vi "run.vi"(8 "error in (no error)":errorcluster, 11 "DataCollectionDL091104Scaffold.lvclass out":refnum<class "DataCollectionDL091104Scaffold.lvclass">) -> (0 "error out":errorcluster, 3 "DataCollectionDL091104Scaffold.lvclass out":refnum<class "DataCollectionDL091104Scaffold.lvclass">)   [LabVIEW 2010, in "DataCollectionDL091104Scaffold.lvclass"]
uses:
  DataCollectionDL091104Scaffold.lvclass
  action_enum.ctl
  DataCollectionDL091104Scaffold.lvclass/DataCollectionDL091104Scaffold.ctl
  GenericDataCollection/GenericDataCollection/GenericDataCollection.lvclass
  common/classes/ErrorController/ErrorController/class_data.vi
  common/classes/ErrorController/ErrorController/ErrorController.lvclass
panel:
  out "last action":T1=enum."initialise"
  out "event loop counter":i32
  out "statechart loop counter":i32=49
  out "error":errorcluster
  in  "play movie?":bool
  out "finished?":bool=TRUE
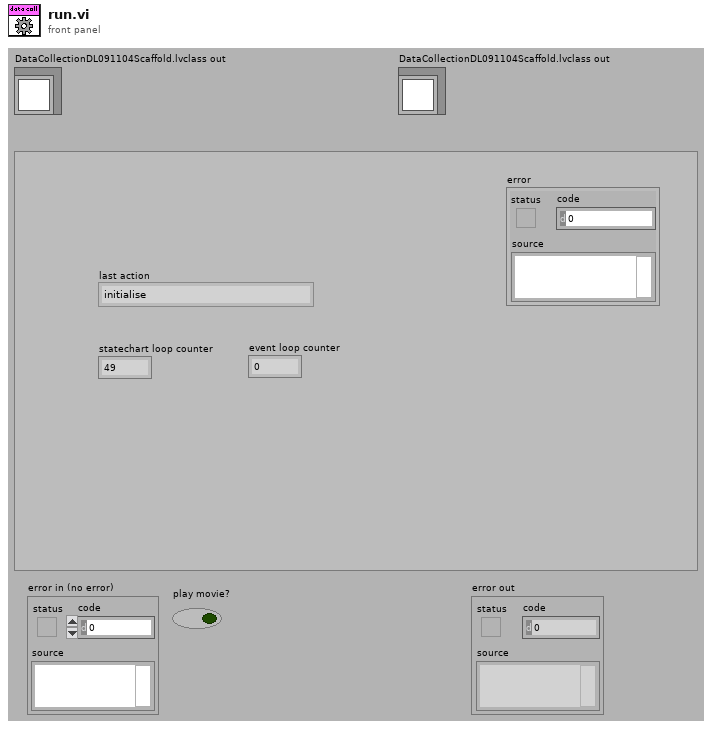
[diagram p1: front panel]
types:
  T1 = typedef "DataCollectionDL091104Scaffold.lvclass/action_enum.ctl" = enum16{"NULL", "initialise", "terminate", "reset", "insert", "save", "register as observer", "sweep finished", "attach observer", "detach observer"}
  T2 = typedef "top-level_component_type_enum.ctl" = enum16{"undefined", "ImagingMode", "ScanHead", "DAQ", "ImageAssembler", "Display", "DataCollection", "Analyser", "Stimulator", "ExperimentController", "Instrument", "Stage"}
  T3 = typedef "main_trigger_enum.ctl" = enum16{"NULL", "initialise", "terminate", "start", "stop", "change objective", "change experimentController", "change imagingMode", "save notebook", "started saving", "finished saving", "expCtr ready", "expCtr missing", "imgMd ready", "imgMd missing", "scanHd ready", "scanHd missing", "DAQ ready", "DAQ missing", "imgAsm ready", "imgAsm missing", "dataColl ready", "dataColl missing", "display ready", "display missing", "analysr ready", "analysr missing", "instrmnt ready", "instrmnt missing", "stimltr ready", "stimltr missing", "stage ready", "stage missing"}
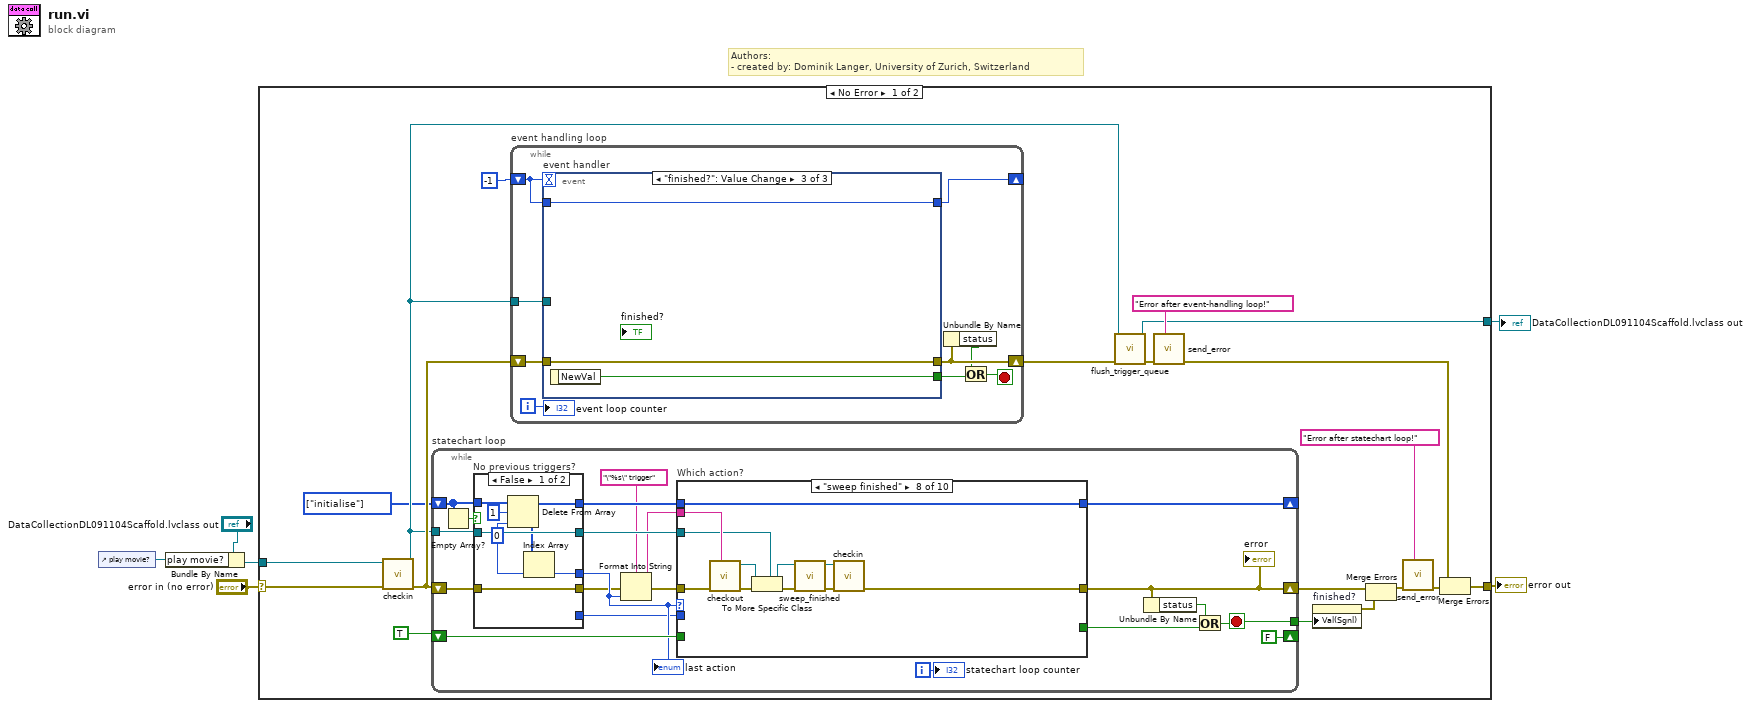
[diagram p0: block diagram]
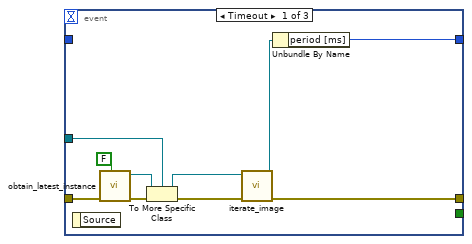
[diagram p2: hidden frame]
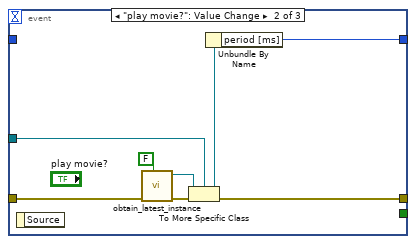
[diagram p3: hidden frame]
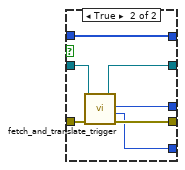
[diagram p4: hidden frame]
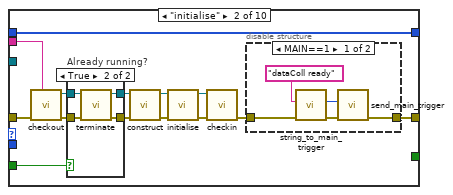
[diagram p6: hidden frame]
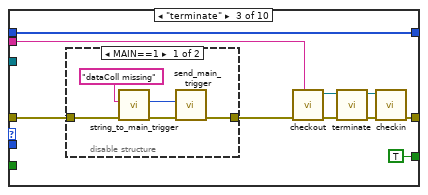
[diagram p9: hidden frame]
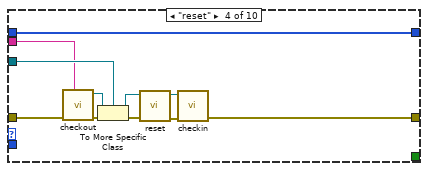
[diagram p11: hidden frame]
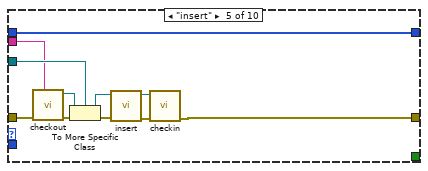
[diagram p12: hidden frame]
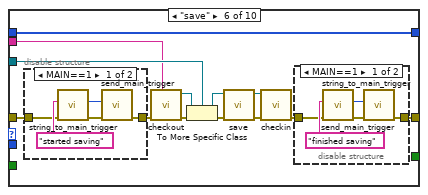
[diagram p13: hidden frame]
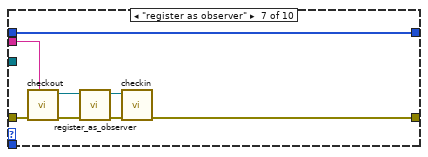
[diagram p16: hidden frame]
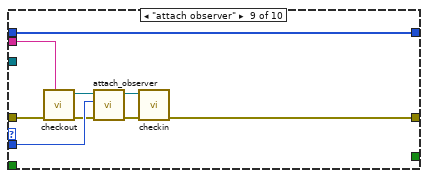
[diagram p17: hidden frame]
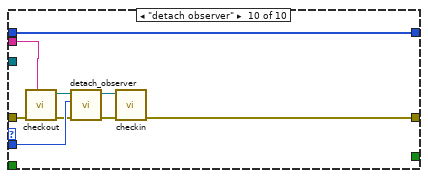
[diagram p18: hidden frame]
diagram:
  # "Authors: \n- created by: Dominik Langer, University of Zurich, Switzerland"
  n1 = control-ref of="play movie?"() -> (w3:refnum<vi>)
  n2 = Bundle By Name(cluster="DataCollectionDL091104Scaffold.lvclass out", "play movie?"=w3) -> (w4:refnum<class "DataCollectionDL091104Scaffold.lvclass">)
  n3 = case shown="No Error" "error in (no error)" {
    selector: "error in (no error)" -> [w7 w220]
    tunnel: [w20 w220] -> w5
    tunnel: [w13 w219] -> w2
    tunnel: w4 -> [w8 w219]
    frame No Error {
      w9 = T1[] [enum."initialise"] items=["NULL", "initialise", "terminate", "reset", "insert", "save", "register as observer", "sweep finished", "attach observer", "detach observer"]
      n4 = call-dynamic "checkin.vi"("error in (no error)"=w7, "GenericDataCollection in"=w8) -> ("error out"=w17:errorcluster, "GenericDataCollection out"=w14:refnum<class "DataCollectionDL091104Scaffold.lvclass">)  [unwired: 8 in]
      n5 = while "statechart loop" {
        shift-right: [FALSE] -> _
        shift-left: TRUE -> [w68]
        tunnel: [w66] -> w23
        tunnel: w14 -> [w73]
        shift-right: [w71] -> w11
        shift-left: w17 -> [w72]
        shift-right: [w62] -> _
        shift-left: w9 -> [w65]
        i -> [w75]
        stop <- w66 stop-if-true
        n6 = Empty Array?(array=w65) -> (empty?=w64:bool)
        n7 = case "No previous triggers?" shown="False" w64 {
          tunnel: w73 -> [w81 w90]
          tunnel: w72 -> [w79 w89]
          tunnel: [w79 w88] -> w59
          tunnel: [w81 w87] -> w67
          tunnel: [w80 w86] -> w61
          tunnel: w65 -> [w83 w85]
          tunnel: [w77 w85] -> w63
          tunnel: [_ w84] -> w56
          frame False {
            w76 = 0 ("index")
            n8 = Delete From Array(array=w83, length=1, index=w76) -> (deleted portion=w78:T1[], array with subset deleted=w77:T1[])
            n9 = Index Array(array=w78, index=w76) -> (element=w80:T1)
          }
          frame True {
            n10 = call-dynamic "fetch_and_translate_trigger.vi"("error in (no error)"=w89, "DataCollectionDL091104Scaffold in"=w90) -> ("error out"=w88:errorcluster, "sender TLC type"=w84:T2, "trigger"=w86:T1, "DataCollectionDL091104Scaffold out"=w87:refnum<class "DataCollectionDL091104Scaffold.lvclass">)  [unwired: 6 in]
          }
        }
        "last action" <- w61
        n11 = Format Into String(format string="\"%s\" trigger", error in=w59, w61) -> (resulting string=w58:string, error out=w60:errorcluster)  [unwired: 1 in]
        n12 = case "Which action?" shown="\"sweep finished\"" w61 {
          tunnel: w60 -> [w92 w98 w122 w145 w149 w160 w187 w197 w207 w216]
          tunnel: [w92 w95 w123 w144 w148 w157 w186 w196 w204 w211] -> w71
          tunnel: [_ _ TRUE _ _ _ _ _ _ _] -> w69
          tunnel: w68 -> [_ w97 _ _ _ _ _ _ _ _]
          tunnel: w67 -> [_ _ _ w143 w150 w163 _ w194 _ _]
          tunnel: w63 -> [w91 w94 w120 w142 w147 w162 w183 w200 w209 w218]
          tunnel: [w91 w94 w120 w142 w147 w162 w183 w200 w209 w218] -> w62
          tunnel: w58 -> [_ w93 w119 w141 w146 w161 w182 w195 w201 w213]
          tunnel: w56 -> [_ _ _ _ _ _ _ _ w208 w217]
          frame "NULL", Default {
          }
          frame "initialise" {
            n13 = call "checkout.vi"("locked by?"=w93, "error in (no error)"=w98) -> ("error out"=w105:errorcluster, "GenericDataCollection out"=w103:refnum<class "GenericDataCollection.lvclass">)  [unwired: 8 in]
            n14 = case "Already running?" shown="True" w97 {
              tunnel: [w114 w118] -> w106
              tunnel: w105 -> [w114 w117]
              tunnel: [w113 w116] -> w104
              tunnel: w103 -> [w113 w115]
              frame False {
              }
              frame True {
                n15 = call-dynamic "terminate.vi"("error in (no error)"=w117, "GenericPlugin in"=w115) -> ("error out"=w118:errorcluster, "GenericPlugin out"=w116:refnum<class "GenericDataCollection.lvclass">)  [unwired: 8 in]
              }
            }
            n16 = call-dynamic "construct.vi"("error in (no error)"=w106, "GenericPlugin in"=w104) -> ("error out"=w101:errorcluster, "GenericPlugin out"=w100:refnum<class "GenericDataCollection.lvclass">)  [unwired: 8 in]
            n17 = call-dynamic "initialise.vi"("error in (no error)"=w101, "GenericPlugin in"=w100) -> ("error out"=w102:errorcluster, "GenericPlugin out"=w99:refnum<class "GenericDataCollection.lvclass">)  [unwired: 8 in]
            n18 = call-dynamic "checkin.vi"("error in (no error)"=w102, "GenericDataCollection in"=w99) -> ("error out"=w96:errorcluster)  [unwired: 8 in, 1 out]
            n19 = disable-structure shown="MAIN==1" {
              disable-tunnel: w96 -> [w109 w112]
              disable-tunnel: [w111 w112] -> w95
              frame condition #0 (active) {
                n20 = call "string_to_main_trigger.vi"("error in (no error)"=w109, "trigger string"="dataColl ready") -> ("error out"=w108:errorcluster, "main trigger"=w107:T3)  [unwired: 8 in]
                n21 = call "send_main_trigger.vi"("error in (no error)"=w108, "trigger"=w107) -> ("error out"=w111:errorcluster)  [unwired: 9 in]
              }
              frame condition #1 {
              }
            }
          }
          frame "terminate" {
            n22 = disable-structure shown="MAIN==1" {
              disable-tunnel: w122 -> [w131 w134]
              disable-tunnel: [w133 w134] -> w121
              frame condition #0 (active) {
                n23 = call "string_to_main_trigger.vi"("error in (no error)"=w131, "trigger string"="dataColl missing") -> ("error out"=w130:errorcluster, "main trigger"=w129:T3)  [unwired: 8 in]
                n24 = call "send_main_trigger.vi"("error in (no error)"=w130, "trigger"=w129) -> ("error out"=w133:errorcluster)  [unwired: 9 in]
              }
              frame condition #1 {
              }
            }
            n25 = call "checkout.vi"("locked by?"=w119, "error in (no error)"=w121) -> ("error out"=w127:errorcluster, "GenericDataCollection out"=w125:refnum<class "GenericDataCollection.lvclass">)  [unwired: 8 in]
            n26 = call-dynamic "terminate.vi"("error in (no error)"=w127, "GenericPlugin in"=w125) -> ("error out"=w126:errorcluster, "GenericPlugin out"=w124:refnum<class "GenericDataCollection.lvclass">)  [unwired: 8 in]
            n27 = call-dynamic "checkin.vi"("error in (no error)"=w126, "GenericDataCollection in"=w124) -> ("error out"=w123:errorcluster)  [unwired: 8 in, 1 out]
          }
          frame "reset" {
            n28 = call "checkout.vi"("locked by?"=w141, "error in (no error)"=w145) -> ("error out"=w137:errorcluster, "GenericDataCollection out"=w140:refnum<class "GenericDataCollection.lvclass">)  [unwired: 8 out]
            n29 = To More Specific Class(target class=w143, reference=w140, error in=w137) -> (specific class reference=w139:refnum<class "DataCollectionDL091104Scaffold.lvclass">, error out=w136:errorcluster)
            n30 = call-dynamic "reset.vi"("error in (no error)"=w136, "DataCollectionDL091104Scaffold in"=w139) -> ("error out"=w135:errorcluster, "DataCollectionDL091104Scaffold out"=w138:refnum<class "DataCollectionDL091104Scaffold.lvclass">)  [unwired: 8 in]
            n31 = call-dynamic "checkin.vi"("error in (no error)"=w135, "GenericDataCollection in"=w138) -> ("error out"=w144:errorcluster)  [unwired: 8 in, 1 out]
          }
          frame "insert" {
            n32 = call "checkout.vi"("locked by?"=w146, "error in (no error)"=w149) -> ("error out"=w155:errorcluster, "GenericDataCollection out"=w156:refnum<class "GenericDataCollection.lvclass">)  [unwired: 8 out]
            n33 = To More Specific Class(target class=w150, reference=w156, error in=w155) -> (specific class reference=w153:refnum<class "DataCollectionDL091104Scaffold.lvclass">, error out=w154:errorcluster)
            n34 = call-dynamic "insert.vi"("error in (no error)"=w154, "DL090215DataCollection in"=w153) -> ("error out"=w152:errorcluster, "DL090215DataCollection out"=w151:refnum<class "DataCollectionDL091104Scaffold.lvclass">)  [unwired: 8 out]
            n35 = call-dynamic "checkin.vi"("error in (no error)"=w152, "GenericDataCollection in"=w151) -> ("error out"=w148:errorcluster)  [unwired: 8 in, 1 out]
          }
          frame "save" {
            n36 = disable-structure shown="MAIN==1" {
              disable-tunnel: w160 -> [w178 w181]
              disable-tunnel: [w180 w181] -> w159
              frame condition #0 (active) {
                n37 = call "string_to_main_trigger.vi"("error in (no error)"=w178, "trigger string"="started saving") -> ("error out"=w177:errorcluster, "main trigger"=w176:T3)  [unwired: 8 in]
                n38 = call "send_main_trigger.vi"("error in (no error)"=w177, "trigger"=w176) -> ("error out"=w180:errorcluster)  [unwired: 9 in]
              }
              frame condition #1 {
              }
            }
            n39 = call "checkout.vi"("locked by?"=w161, "error in (no error)"=w159) -> ("error out"=w166:errorcluster, "GenericDataCollection out"=w169:refnum<class "GenericDataCollection.lvclass">)  [unwired: 8 out]
            n40 = To More Specific Class(target class=w163, reference=w169, error in=w166) -> (specific class reference=w167:refnum<class "DataCollectionDL091104Scaffold.lvclass">, error out=w165:errorcluster)
            n41 = call-dynamic "save.vi"("error in (no error)"=w165, "DL090215DataCollection in"=w167) -> ("error out"=w164:errorcluster, "DL090215DataCollection out"=w168:refnum<class "DataCollectionDL091104Scaffold.lvclass">)  [unwired: 8 out]
            n42 = call-dynamic "checkin.vi"("error in (no error)"=w164, "GenericDataCollection in"=w168) -> ("error out"=w158:errorcluster)  [unwired: 8 in, 1 out]
            n43 = disable-structure shown="MAIN==1" {
              disable-tunnel: w158 -> [w172 w175]
              disable-tunnel: [w174 w175] -> w157
              frame condition #0 (active) {
                n44 = call "string_to_main_trigger.vi"("error in (no error)"=w172, "trigger string"="finished saving") -> ("error out"=w171:errorcluster, "main trigger"=w170:T3)  [unwired: 8 in]
                n45 = call "send_main_trigger.vi"("error in (no error)"=w171, "trigger"=w170) -> ("error out"=w174:errorcluster)  [unwired: 9 in]
              }
              frame condition #1 {
              }
            }
          }
          frame "register as observer" {
            n46 = call "checkout.vi"("locked by?"=w182, "error in (no error)"=w187) -> ("error out"=w184:errorcluster, "GenericDataCollection out"=w189:refnum<class "GenericDataCollection.lvclass">)  [unwired: 8 in]
            n47 = call-dynamic "register_as_observer.vi"("error in (no error)"=w184, "GenericToplevelComponent in"=w189) -> ("error out"=w185:errorcluster, "GenericToplevelComponent out"=w188:refnum<class "GenericDataCollection.lvclass">)  [unwired: 8 in]
            n48 = call-dynamic "checkin.vi"("error in (no error)"=w185, "GenericDataCollection in"=w188) -> ("error out"=w186:errorcluster)  [unwired: 8 in, 1 out]
          }
          frame "sweep finished" {
            n49 = call "checkout.vi"("locked by?"=w195, "error in (no error)"=w197) -> ("error out"=w192:errorcluster, "GenericDataCollection out"=w193:refnum<class "GenericDataCollection.lvclass">)  [unwired: 8 in]
            n50 = To More Specific Class(target class=w194, reference=w193, error in=w192) -> (specific class reference=w190:refnum<class "DataCollectionDL091104Scaffold.lvclass">, error out=w191:errorcluster)
            n51 = call-dynamic "sweep_finished.vi"("error in (no error)"=w191, "DataCollectionDL091104Scaffold in"=w190) -> ("error out"=w199:errorcluster, "DataCollectionDL091104Scaffold out"=w198:refnum<class "DataCollectionDL091104Scaffold.lvclass">)  [unwired: 8 in]
            n52 = call-dynamic "checkin.vi"("error in (no error)"=w199, "GenericDataCollection in"=w198) -> ("error out"=w196:errorcluster)  [unwired: 8 in, 1 out]
          }
          frame "attach observer" {
            n53 = call "checkout.vi"("locked by?"=w201, "error in (no error)"=w207) -> ("error out"=w206:errorcluster, "GenericDataCollection out"=w203:refnum<class "GenericDataCollection.lvclass">)  [unwired: 8 in]
            n54 = call-dynamic "attach_observer.vi"("error in (no error)"=w206, "top-level component type"=w208, "GenericToplevelComponent in"=w203) -> ("error out"=w205:errorcluster, "GenericToplevelComponent out"=w202:refnum<class "GenericDataCollection.lvclass">)  [unwired: 7 in]
            n55 = call-dynamic "checkin.vi"("error in (no error)"=w205, "GenericDataCollection in"=w202) -> ("error out"=w204:errorcluster)  [unwired: 8 in, 1 out]
          }
          frame "detach observer" {
            n56 = call "checkout.vi"("locked by?"=w213, "error in (no error)"=w216) -> ("error out"=w215:errorcluster, "GenericDataCollection out"=w214:refnum<class "GenericDataCollection.lvclass">)  [unwired: 8 in]
            n57 = call-dynamic "detach_observer.vi"("error in (no error)"=w215, "top-level component type"=w217, "GenericToplevelComponent in"=w214) -> ("error out"=w212:errorcluster, "GenericToplevelComponent out"=w210:refnum<class "GenericDataCollection.lvclass">)  [unwired: 7 in]
            n58 = call-dynamic "checkin.vi"("error in (no error)"=w212, "GenericDataCollection in"=w210) -> ("error out"=w211:errorcluster)  [unwired: 8 in, 1 out]
          }
        }
        "error" <- w71
        n59 = Unbundle By Name(w71) -> ("status"=w70:bool)
        n60 = Or(x=w70, y=w69) -> (x .or. y?=w66:bool)
        "statechart loop counter" <- w75
      }
      n61 = while "event handling loop" {
        shift-right: [w33] -> _
        shift-left: -1 -> [w34]
        tunnel: w14 -> [w31]
        shift-right: [w29] -> w16
        shift-left: w17 -> [w32]
        i -> [w30]
        stop <- w26 stop-if-true
        n62 = event "event handler" shown="[2] \"finished?\": Value Change" {
          selector: _ -> [_ _ _]
          dyn-events: _ -> [_ _ _]
          timeout: w34 -> [_ _ _]
          tunnel: w34 -> [_ _ w55]
          tunnel: [w39 w45 w55] -> w33
          tunnel: w32 -> [w41 w48 w54]
          tunnel: [w37 w47 w54] -> w29
          tunnel: [_ _ w53] -> w28
          tunnel: w31 -> [w42 w49 _]
          event Timeout {
            n63 = event-data() -> ()  [unwired: 2 out]
            n64 = call "obtain_latest_instance.vi"("quick, but maybe outdated?"=FALSE, "error in (no error)"=w41) -> ("error out"=w44:errorcluster, "GenericDataCollection out"=w43:refnum<class "GenericDataCollection.lvclass">)  [unwired: 8 in]
            n65 = To More Specific Class(target class=w42, reference=w43, error in=w44) -> (specific class reference=w36:refnum<class "DataCollectionDL091104Scaffold.lvclass">, error out=w38:errorcluster)
            n66 = call-dynamic "iterate_image.vi"("error in (no error)"=w38, "DL090215DataCollection in"=w36) -> ("error out"=w37:errorcluster, "DL090215DataCollection out"=w35:refnum<class "DataCollectionDL091104Scaffold.lvclass">)  [unwired: 8 in]
            n67 = Unbundle By Name(w35) -> ("period [ms]"=w39:i32)
          }
          event "play movie?": Value Change {
            n68 = event-data() -> ()  [unwired: 2 out]
            n69 = call "obtain_latest_instance.vi"("quick, but maybe outdated?"=FALSE, "error in (no error)"=w48) -> ("error out"=w50:errorcluster, "GenericDataCollection out"=w51:refnum<class "GenericDataCollection.lvclass">)  [unwired: 8 in]
            n70 = To More Specific Class(target class=w49, reference=w51, error in=w50) -> (specific class reference=w46:refnum<class "DataCollectionDL091104Scaffold.lvclass">, error out=w47:errorcluster)
            n71 = Unbundle By Name(w46) -> ("period [ms]"=w45:i32)
          }
          event "finished?": Value Change {
            n72 = event-data() -> ("NewVal"=w53:bool)  [unwired: 1 out]
          }
        }
        n73 = Unbundle By Name(w29) -> ("status"=w27:bool)
        n74 = Or(x=w27, y=w28) -> (x .or. y?=w26:bool)
        "event loop counter" <- w30
      }
      n75 = call-dynamic "flush_trigger_queue.vi"("error in (no error)"=w16, "GenericToplevelComponent in"=w14) -> ("error out"=w15:errorcluster, "GenericToplevelComponent out"=w13:refnum<class "DataCollectionDL091104Scaffold.lvclass">)  [unwired: 8 in]
      n76 = call "send_error.vi"("additional message"="Error after event-handling loop!", "error in (no error)"=w15) -> ("error out"=w22:errorcluster)  [unwired: 9 in]
      n77 = property on="finished?" class="Bool (strict)"("Val(Sgnl)"=w23) -> (error out=w12:errorcluster)  [unwired: 2 in, 1 out]
      n78 = Merge Errors(w11, w12) -> (w10:errorcluster)
      n79 = call "send_error.vi"("additional message"="Error after statechart loop!", "error in (no error)"=w10) -> ("error out"=w19:errorcluster)  [unwired: 9 in]
      n80 = Merge Errors(w22, w19) -> (w20:errorcluster)
    }
    frame Error {
    }
  }
  "error out" <- w5
  "DataCollectionDL091104Scaffold.lvclass out" <- w2
